vi "Robot FPGA Utility for screenshots.vi"() -> ()   [LabVIEW 2014]
doc: "This FPGA VI defines the functionality that is needed for the C terminal connector for the myRIO sheepdog robot project. It provides two PWM outputs, two single-line counters (for the Hall effect encoders), and digital IO needed to command the motors. It also determines a measure of the derivative of the encoder counter lines (proportional to wheel speed)."
uses:
  <vilib>/Platform/TimedLoop/XDataNode/XDataNode.xnode
  <vilib>/Platform/TimedLoop/XDataNode/nitl_modes.ctl
  <vilib>/Platform/TimedLoop/XDataNode/XDNodeRunTimeDep.lvlib
  <vilib>/Platform/TimedLoop/XDataNode/wakeup.ctl
  <vilib>/Platform/TimedLoop/XDataNode/timing_clust.ctl
  <vilib>/eio/EIONode/EIONode.xnode
  <vilib>/rvi/eio/common/nirviEmuTemplateMethod_errors.vi
  <vilib>/eio/EIOMethodNode/EIOMethodNode.xnode
panel:
  in  "Motor Dir 2":bool
  in  "Motor Dir 1":bool
  out "Encoder 2 Period":u32
  out "Encoder 2 Position":i16
  out "Encoder 1 Period":u32
  out "Encoder 1 Position":i16
  in  "Reset Encoder 2":bool
  in  "Reset Encoder 1":bool
  in  "Duty Cycle Divisor":i16=30000
  in  "Duty Cycle 2":i16
  in  "Duty Cycle 1":i16
  out "SYS.RDY":bool=TRUE
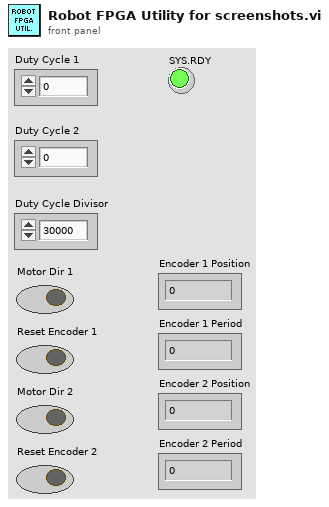
[diagram p1: front panel]
types:
  T1 = typedef "XDNodeRunTimeDep.lvlib/timing_clust.ctl" = cluster{"Expected End [f-1]":u64, "Actual End [f-1]":u64, "Finished Late? [f-1]":bool, "Expected End [i-1]":u64, "Actual End [i-1]":u64, "Finished Late? [i-1]":bool, "Expected Start [i]":u64, "Actual Start [i]":u64, "Expected Start [f]":u64, "Actual Start [f]":u64, "Source Name":string, "Structure Name":string, "Period":i64, "Deadline":i64, "Offset":i64, "Start":i64, "Priority":i32, "Timeout":i32, "Mode":T2, "Wakeup Reason":T3, "Error":errorcluster, "Source Type":string, "Secondary Source Type":string, "Global End Time":u64, "Global Start Time":u64, "Frame Duration":u64, "Iteration Duration":u64, "Assigned CPU":i32, "I/O Scan Engine Mode":u32}
  T2 = typedef "XDNodeRunTimeDep.lvlib/nitl_modes.ctl" = enum32{"No Change", "Process missed periods, maintain original phase", "Discard missed periods, maintain original phase", "Process missed periods, ignore original phase", "Discard missed periods, ignore original phase"}
  T3 = typedef "XDNodeRunTimeDep.lvlib/wakeup.ctl" = enum32{"Normal", "Aborted", "Asynchronous wakeup", "Timing source error", "Timed loop error", "Timeout"}
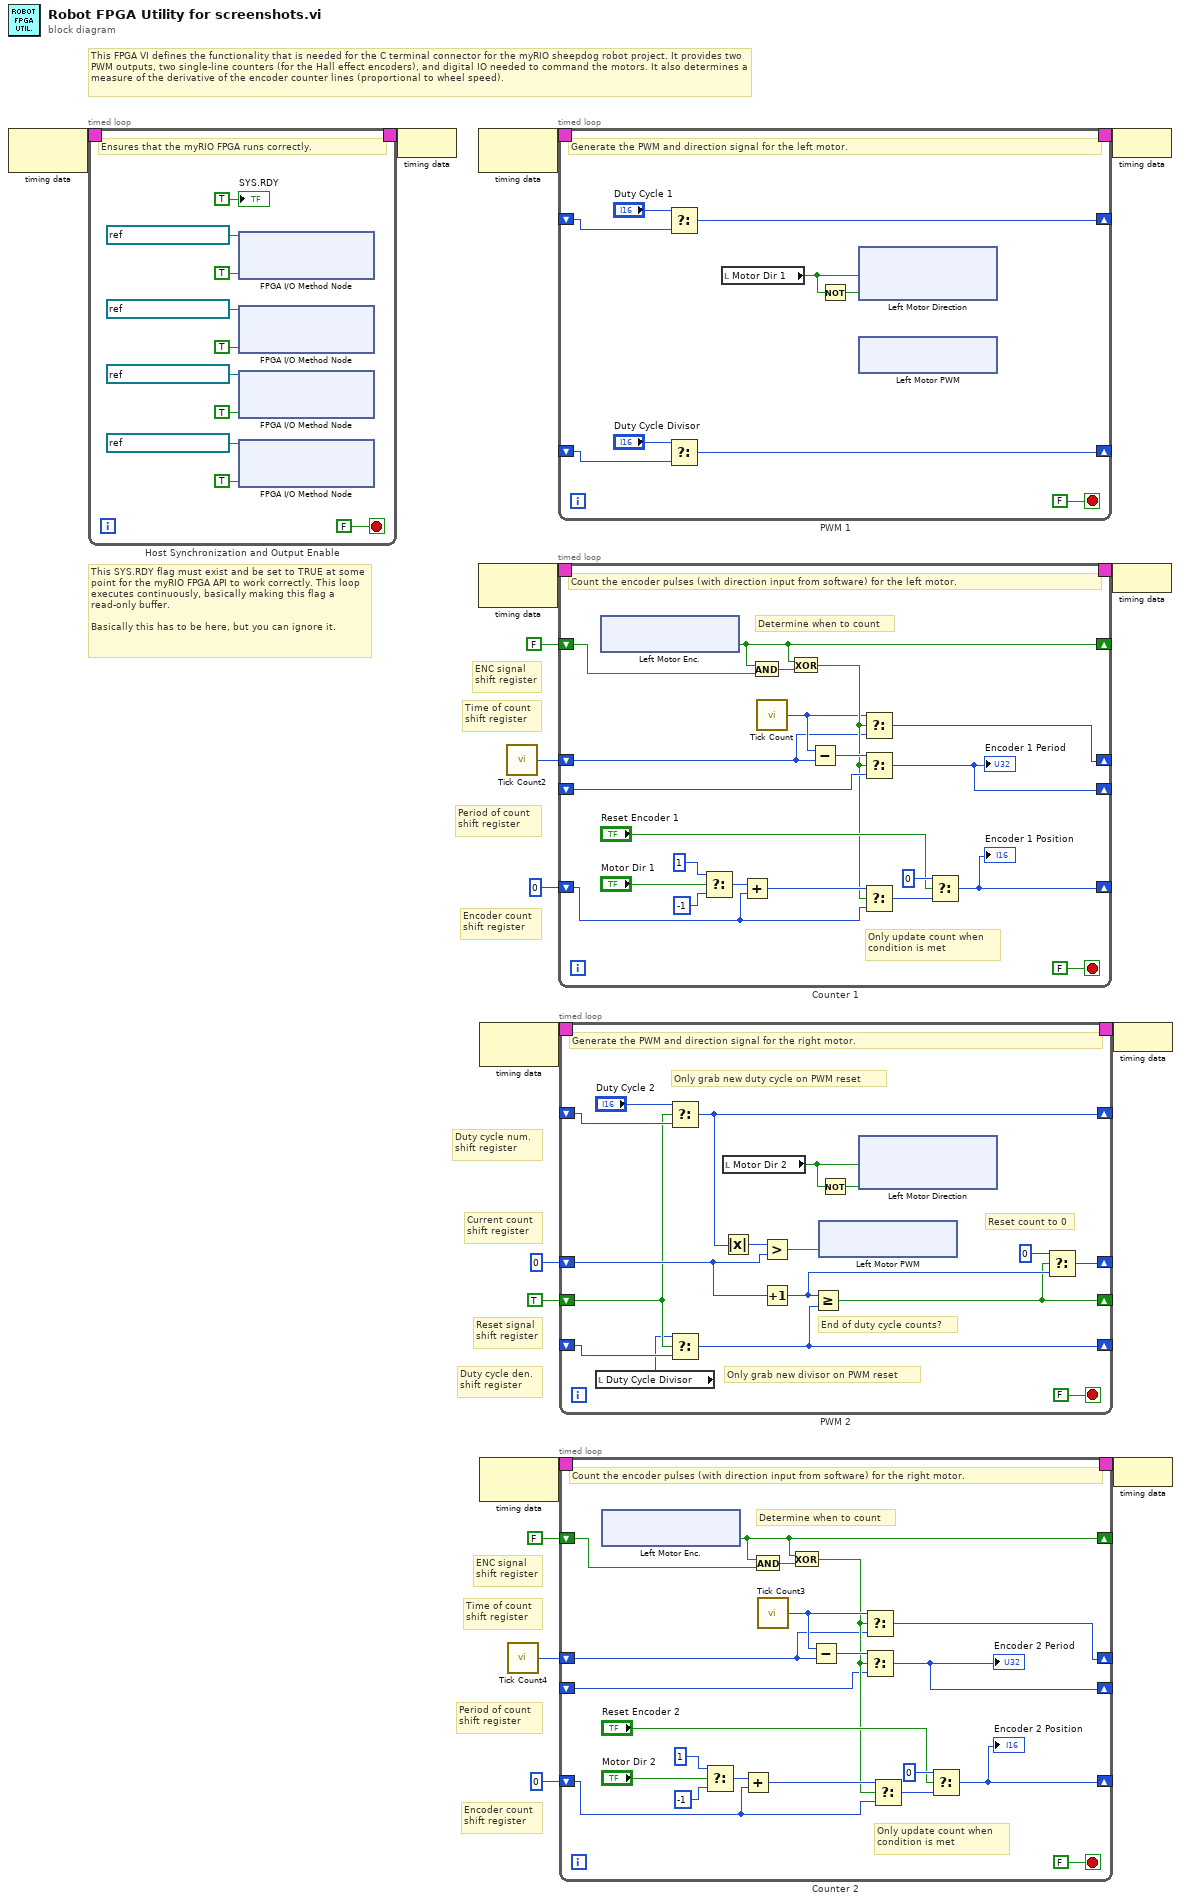
[diagram p0: block diagram]
diagram:
  # "Period of count\nshift register"
  # "Period of count\nshift register"
  # "This SYS.RDY flag must exist and be set to TRUE at some point for the myRIO FPGA API to work correctly. This loop executes continuously, basically making this flag a read-only buffer.\n\nBasically this has to be here, but you can ignore it."
  # "Time of count\nshift register"
  # "Encoder count\nshift register"
  # "ENC signal\nshift register"
  # "Current count\nshift register"
  # "Reset signal\nshift register"
  # "Duty cycle den.\nshift register"
  # "Duty cycle num.\nshift register"
  # "Time of count\nshift register"
  # "Encoder count\nshift register"
  # "ENC signal\nshift register"
  # "This FPGA VI defines the functionality that is needed for the C terminal connector for the myRIO sheepdog robot project. It provides two PWM outputs, two single-line counters (for the Hall effect encoders), and digital IO needed to command the motors. It also determines a measure of the derivative of the encoder counter lines (proportional to wheel speed)."
  n1 = node-c288() -> (w2:T1)  [unwired: 1 in]
  n2 = timed-loop "Host Synchronization and Output Enable" {
    timing: w2 -> [_]
    timing-out: [_] -> w1
    stop <- FALSE stop-if-true
    # "Ensures that the myRIO FPGA runs correctly."
    n3 = xnode "FPGA I/O Method Node"("FPGA I/O In"=refnum<k21> "ConnectorC/DIO1", "Enable"=TRUE) -> ()  [unwired: 1 out]
    n4 = xnode "FPGA I/O Method Node"("FPGA I/O In"=refnum<k21> "ConnectorC/DIO3", "Enable"=TRUE) -> ()  [unwired: 1 out]
    n5 = xnode "FPGA I/O Method Node"("FPGA I/O In"=refnum<k21> "ConnectorC/DIO5", "Enable"=TRUE) -> ()  [unwired: 1 out]
    n6 = xnode "FPGA I/O Method Node"("FPGA I/O In"=refnum<k21> "ConnectorC/DIO7", "Enable"=TRUE) -> ()  [unwired: 1 out]
    "SYS.RDY" <- TRUE
  }
  n7 = node-c288(w1) -> ()
  n8 = node-c288() -> (w18:T1)  [unwired: 1 in]
  n9 = node-c288() -> (w16:T1)  [unwired: 1 in]
  n10 = node-c288() -> (w11:T1)  [unwired: 1 in]
  n11 = node-c288() -> (w9:T1)  [unwired: 1 in]
  n12 = call "Tick Count2"() -> ("Tick Count(Ticks)"=w14:u32)
  n13 = call "Tick Count4"() -> ("Tick Count(Ticks)"=w5:u32)
  n14 = timed-loop "PWM 1" {
    timing: w18 -> [_]
    timing-out: [_] -> w17
    shift-right: [w37] -> _
    shift-left: _ -> [w38]
    shift-right: [w34] -> _
    shift-left: _ -> [w33]
    stop <- FALSE stop-if-true
    # "Generate the PWM and direction signal for the left motor."
    n15 = Select(t="Duty Cycle 1", f=w38) -> (s? t:f=w37:i16)  [unwired: 1 in]
    n16 = Select(t="Duty Cycle Divisor", f=w33) -> (s? t:f=w34:i16)  [unwired: 1 in]
    n17 = local read "Motor Dir 1"() -> (w31:bool)
    n18 = Not(x=w31) -> (.not. x?=w32:bool)
    n19 = xnode "Left Motor Direction"("ConnectorC/DIO0"=w31, "ConnectorC/DIO1"=w32) -> ()  [unwired: 2 in, 2 out]
    n20 = xnode "Left Motor PWM"() -> ()  [unwired: 2 in, 1 out]
  }
  n21 = timed-loop "Counter 1" {
    timing: w16 -> [_]
    timing-out: [_] -> w15
    shift-right: [w53] -> _
    shift-left: i16 0 ("t") -> [w54]
    shift-right: [w50] -> _
    shift-left: FALSE ("ConnectorC/DIO2") -> [w52]
    shift-right: [w42] -> _
    shift-left: w14 -> [w43]
    shift-right: [w46] -> _
    shift-left: _ -> [w47]
    stop <- FALSE stop-if-true
    # "Determine when to count"
    # "Only update count when\ncondition is met"
    # "Count the encoder pulses (with direction input from software) for the left motor."
    n22 = xnode "Left Motor Enc."() -> ("ConnectorC/DIO2"=w50:bool)  [unwired: 1 in, 1 out]
    n23 = Select(t=i16 1, s="Motor Dir 1", f=i16 -1) -> (s? t:f=w59:i16)
    n24 = Add(x=w59, y=w54) -> (x+y=w58:i16)
    n25 = And(x=w50, y=w52) -> (x .and. y?=w51:bool)
    n26 = call "Tick Count"() -> ("Tick Count(Ticks)"=w44:u32)
    n27 = Exclusive Or(1:w51, 2:w50) -> (0:w45:bool)
    n28 = Subtract(x=w44, y=w43) -> (x-y=w49:u32)
    n29 = Select(t=w44, s=w45, f=w43) -> (s? t:f=w42:u32)
    n30 = Select(t=w49, s=w45, f=w47) -> (s? t:f=w46:u32)
    "Encoder 1 Period" <- w46
    n31 = Select(t=w58, s=w45, f=w54) -> (s? t:f=w57:i16)
    n32 = Select(t=i16 0, s="Reset Encoder 1", f=w57) -> (s? t:f=w53:i16)
    "Encoder 1 Position" <- w53
  }
  n33 = timed-loop "PWM 2" {
    timing: w11 -> [_]
    timing-out: [_] -> w10
    shift-right: [w80] -> _
    shift-left: _ -> [w81]
    shift-right: [w74] -> _
    shift-left: i16 0 -> [w77]
    shift-right: [w72] -> _
    shift-left: TRUE -> [w71]
    shift-right: [w70] -> _
    shift-left: _ -> [w69]
    stop <- FALSE stop-if-true
    # "Only grab new divisor on PWM reset"
    # "End of duty cycle counts?"
    # "Reset count to 0"
    # "Only grab new duty cycle on PWM reset"
    # "Generate the PWM and direction signal for the right motor."
    n34 = local read "Duty Cycle Divisor"() -> (w67:i16)
    n35 = Select(t="Duty Cycle 2", s=w71, f=w81) -> (s? t:f=w80:i16)
    n36 = Select(t=w67, s=w71, f=w69) -> (s? t:f=w70:i16)
    n37 = local read "Motor Dir 2"() -> (w66:bool)
    n38 = Absolute Value(x=w80) -> (abs(x)=w79:i16)
    n39 = Greater?(x=w79, y=w77) -> (0:w78:bool)
    n40 = Increment(x=w77) -> (x+1=w76:i16)
    n41 = Greater Or Equal?(x=w76, y=w70) -> (x >= y?=w72:bool)
    n42 = xnode "Left Motor PWM"("ConnectorC/DIO7"=w78) -> ()  [unwired: 1 in, 1 out]
    n43 = Not(x=w66) -> (.not. x?=w65:bool)
    n44 = xnode "Left Motor Direction"("ConnectorC/DIO4"=w66, "ConnectorC/DIO5"=w65) -> ()  [unwired: 2 in, 2 out]
    n45 = Select(t=i16 0, s=w72, f=w76) -> (s? t:f=w74:i16)
  }
  n46 = timed-loop "Counter 2" {
    timing: w9 -> [_]
    timing-out: [_] -> w8
    shift-right: [w93] -> _
    shift-left: i16 0 ("t") -> [w98]
    shift-right: [w95] -> _
    shift-left: FALSE ("ConnectorC/DIO2") -> [w97]
    shift-right: [w84] -> _
    shift-left: w5 -> [w87]
    shift-right: [w86] -> _
    shift-left: _ -> [w85]
    stop <- FALSE stop-if-true
    # "Determine when to count"
    # "Only update count when\ncondition is met"
    # "Count the encoder pulses (with direction input from software) for the right motor."
    n47 = xnode "Left Motor Enc."() -> ("ConnectorC/DIO6"=w95:bool)  [unwired: 1 in, 1 out]
    n48 = Select(t=i16 1, s="Motor Dir 2", f=i16 -1) -> (s? t:f=w102:i16)
    n49 = Add(x=w102, y=w98) -> (x+y=w101:i16)
    n50 = And(x=w95, y=w97) -> (x .and. y?=w96:bool)
    n51 = call "Tick Count3"() -> ("Tick Count(Ticks)"=w89:u32)
    n52 = Exclusive Or(1:w96, 2:w95) -> (0:w88:bool)
    n53 = Subtract(x=w89, y=w87) -> (x-y=w90:u32)
    n54 = Select(t=w89, s=w88, f=w87) -> (s? t:f=w84:u32)
    n55 = Select(t=w90, s=w88, f=w85) -> (s? t:f=w86:u32)
    "Encoder 2 Period" <- w86
    n56 = Select(t=w101, s=w88, f=w98) -> (s? t:f=w100:i16)
    n57 = Select(t=i16 0, s="Reset Encoder 2", f=w100) -> (s? t:f=w93:i16)
    "Encoder 2 Position" <- w93
  }
  n58 = node-c288(w17) -> ()
  n59 = node-c288(w15) -> ()
  n60 = node-c288(w10) -> ()
  n61 = node-c288(w8) -> ()
